vi "Get Op State.vi"(8 "error in (no error)":errorcluster) -> (0 "error out":errorcluster, 2 "operation (meas. mode)":T1=enum."Measurement mode")   [LabVIEW 2015]
doc: "Returns the current operation state of the WLM.\n\n0= Measurement off\n1= Adjustment mode\n2= measurement mode"
uses:
  HighFinesse WS5/Control typedefs.llb/Measurement Mode.ctl
  HighFinesse WS5/wlmData.dll
  HighFinesse WS5/HighFinesse WS5.lvlib
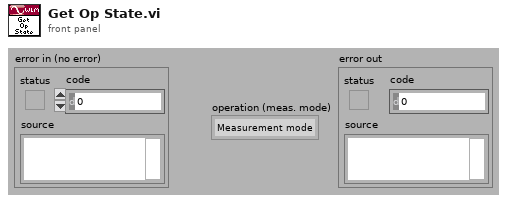
[diagram p1: front panel]
types:
  T1 = typedef "HighFinesse WS5.lvlib/Measurement Mode.ctl" = enum16{"Measurement off", "Adjustment mode", "Measurement mode"}
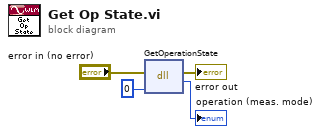
[diagram p0: block diagram]
diagram:
  n1 = dll-call lib="C:/LabVIEW-programs-dev/Instruments/Wavelength meter/HighFinesse WS5/wlmData.dll" fn="GetOperationState"(error in="error in (no error)", "Op"=u8 0) -> (error out=→"error out":errorcluster, "return type"=→"operation (meas. mode)":u16)  [unwired: 3 in, 1 out]
